vi "Read Configuration and Measurements.vi"(8 "error in (no error)":errorcluster, 11 "MKS MW in":refnum<class "PL MKS MW.lvclass">) -> (0 "error out":errorcluster, 2 "configuration and measurements":T1 {"preset index" items=["0", "1", "2", "3", "4", "5", "6", "7", "8", "9", "A", "B", "C"]; "control mode" items=["manual"=1, "analog"=2, "auto"=3]}, 3 "MKS MW out":refnum<class "PL MKS MW.lvclass">)   [LabVIEW 2015, in "PL MKS MW.lvclass"]
doc: "Reads DC bias voltage, peak-to-peak voltage, C1 and C2 capacitor positions, control mode and index of preset capacitor values."
uses:
  PL MKS MW.lvclass
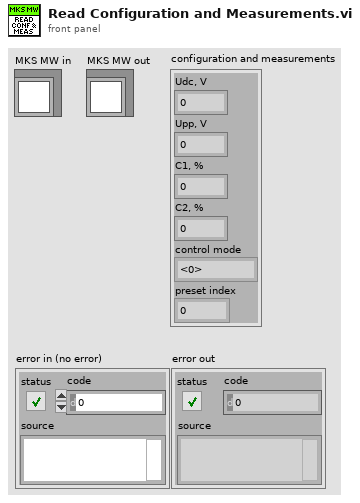
[diagram p1: front panel]
types:
  T1 = cluster{"Udc, V":u16, "Upp, V":u16, "C1, %":u8, "C2, %":u8, "control mode":u16, "preset index":u8}
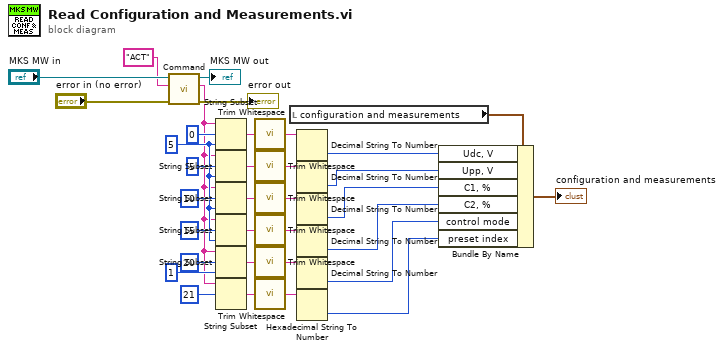
[diagram p0: block diagram]
diagram:
  w24 = 5 ("length (rest)")
  n1 = call "Command.vi"("error in (no error)"="error in (no error)", "command"="ACT", "MKS MW in"="MKS MW in") -> ("error out"=→"error out":errorcluster, "response data"=w17:string, "MKS MW out"=→"MKS MW out":refnum<class "PL MKS MW.lvclass">)  [unwired: 6 in]
  n2 = String Subset(string=w17, offset (0)=0, length (rest)=w24) -> (substring=w23:string)
  n3 = String Subset(string=w17, offset (0)=5, length (rest)=w24) -> (substring=w21:string)
  n4 = String Subset(string=w17, offset (0)=10, length (rest)=w24) -> (substring=w20:string)
  n5 = String Subset(string=w17, offset (0)=15, length (rest)=w24) -> (substring=w19:string)
  n6 = String Subset(string=w17, offset (0)=20, length (rest)=1 ("length (rest)")) -> (substring=w22:string)
  n7 = String Subset(string=w17, offset (0)=21) -> (substring=w15:string)  [unwired: 1 in]
  n8 = call <vilib>:"Trim Whitespace.vi"("string"=w23) -> ("trimmed string"=w14:string)  [unwired: 1 in]
  n9 = call <vilib>:"Trim Whitespace.vi"("string"=w21) -> ("trimmed string"=w12:string)  [unwired: 1 in]
  n10 = call <vilib>:"Trim Whitespace.vi"("string"=w20) -> ("trimmed string"=w11:string)  [unwired: 1 in]
  n11 = call <vilib>:"Trim Whitespace.vi"("string"=w19) -> ("trimmed string"=w10:string)  [unwired: 1 in]
  n12 = call <vilib>:"Trim Whitespace.vi"("string"=w22) -> ("trimmed string"=w13:string)  [unwired: 1 in]
  n13 = call <vilib>:"Trim Whitespace.vi"("string"=w15) -> ("trimmed string"=w9:string)  [unwired: 1 in]
  n14 = local read "configuration and measurements"() -> (w8:T1)
  n15 = Decimal String To Number(string=w14) -> (number=w7:i32)  [unwired: 2 in, 1 out]
  n16 = Decimal String To Number(string=w12) -> (number=w6:i32)  [unwired: 2 in, 1 out]
  n17 = Decimal String To Number(string=w11) -> (number=w5:i32)  [unwired: 2 in, 1 out]
  n18 = Decimal String To Number(string=w10) -> (number=w4:i32)  [unwired: 2 in, 1 out]
  n19 = Decimal String To Number(string=w13) -> (number=w3:i32)  [unwired: 2 in, 1 out]
  n20 = Hexadecimal String To Number(string=w9) -> (number=w2:u32)  [unwired: 2 in, 1 out]
  n21 = Bundle By Name(cluster=w8, "Udc, V"=w7, "Upp, V"=w6, "C1, %"=w5, "C2, %"=w4, "control mode"=w3, "preset index"=w2) -> (→"configuration and measurements":T1)
